vi "CD Shared lvlib.vi"(9 "Action":T1) -> (1 "Output":string)   [LabVIEW 2020, in "NIVS_Consolidated_CDW_MetaDataObj.lvclass"]
doc: "Constants, which are necessary for the <B>CD Shared library</B> in the generated custom device project."
uses:
  NIVS_Consolidated_CDW_MetaDataObj.lvclass
  CD Shared lvlib.ctl
  Common.ctl
  Common.vi
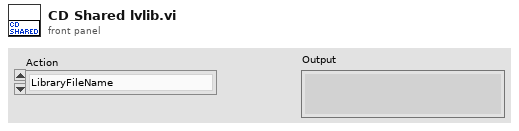
[diagram p1: front panel]
types:
  T1 = typedef "NIVS_Consolidated_CDW_MetaDataObj.lvclass/CD Shared lvlib.ctl" = enum16{"LibraryFileName", "LibraryFolderName", "ConstantsVI.VIPathAndName", "Shared.FolderName", "Shared.Types.FolderName", "Shared.Constants.VIName", "Shared.Constants.VITemplateName", "Shared.Constants.VITemplatePathAndName", "Shared.CompiledSettings.RelativePath", "Shared.Constants.RelativePath", "Shared.CompiledSettings.Name", "Shared.CompiledSettings.Name.NoExtension", "Shared.CompiledSettings.ClusterName"}
  T2 = typedef "NIVS_Consolidated_CDW_MetaDataObj.lvclass/Common.ctl" = enum16{"ProjectName", "TemplatesFolderName", "PPLTemplatesFolderName", "ProjectTemplatePathAndName", "ProjectPPLTemplatePathAndName", "TimingAndSyncFolderName", "CustomDeviceFolderName", "PathToTemplates", "PathToPPLTemplates", "PathToExplorerPPLTemplates", "PathToEnginePPLTemplates", "PathToConfigurationFile", "ProjectConfigurationName"}
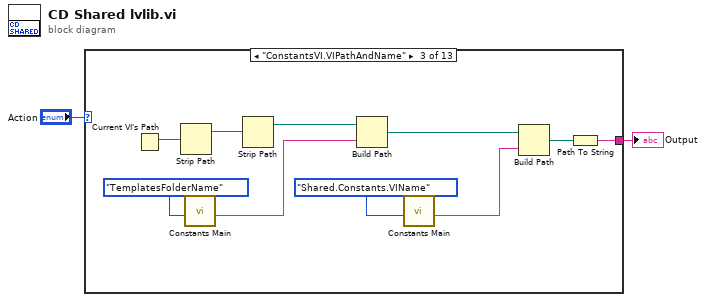
[diagram p0: block diagram]
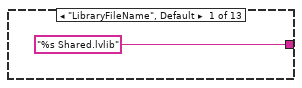
[diagram p2: hidden frame]
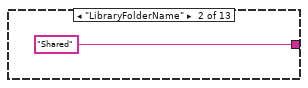
[diagram p3: hidden frame]
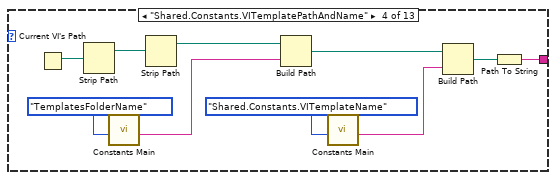
[diagram p4: hidden frame]
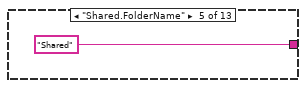
[diagram p5: hidden frame]
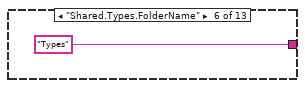
[diagram p6: hidden frame]
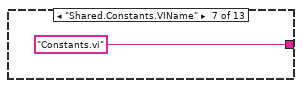
[diagram p7: hidden frame]
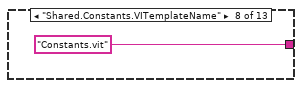
[diagram p8: hidden frame]
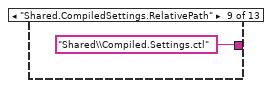
[diagram p9: hidden frame]
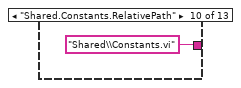
[diagram p10: hidden frame]
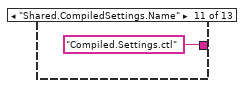
[diagram p11: hidden frame]
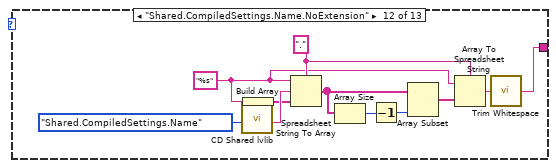
[diagram p12: hidden frame]
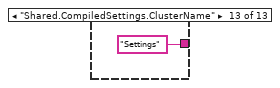
[diagram p13: hidden frame]
diagram:
  n1 = case shown="\"ConstantsVI.VIPathAndName\"" "Action" {
    tunnel: ["%s Shared.lvlib" "Shared" w14 w24 "Shared" "Types" "Constants.vi" "Constants.vit" "Shared\\Compiled.Settings.ctl" ("name or relative path") "Shared\\Constants.vi" ("name or relative path") "Compiled.Settings.ctl" ("name or relative path") w32 "Settings" ("name or relative path")] -> w2
    frame "LibraryFileName", Default {
    }
    frame "LibraryFolderName" {
    }
    frame "ConstantsVI.VIPathAndName" {
      n2 = Current VI's Path() -> (path=w7:path)
      n3 = Strip Path(path=w7) -> (stripped path=w6:path)  [unwired: 1 out]
      n4 = call-poly "Constants Main.vi"("Action"=Common."TemplatesFolderName") -> ("Output"=w12:string)  [unwired: 10 in]
      n5 = Strip Path(path=w6) -> (stripped path=w5:path)  [unwired: 1 out]
      n6 = Build Path(base path=w5, name or relative path=w12) -> (appended path=w11:path)
      n7 = call-poly "Constants Main.vi"("Action"=CD_Shared_lvlib."Shared.Constants.VIName") -> ("Output"=w8:string)  [unwired: 10 in]
      n8 = Build Path(base path=w11, name or relative path=w8) -> (appended path=w10:path)
      n9 = Path To String(path=w10) -> (string=w14:string)
    }
    frame "Shared.Constants.VITemplatePathAndName" {
      n10 = Current VI's Path() -> (path=w17:path)
      n11 = Strip Path(path=w17) -> (stripped path=w16:path)  [unwired: 1 out]
      n12 = call-poly "Constants Main.vi"("Action"=Common."TemplatesFolderName") -> ("Output"=w22:string)  [unwired: 10 in]
      n13 = Strip Path(path=w16) -> (stripped path=w15:path)  [unwired: 1 out]
      n14 = Build Path(base path=w15, name or relative path=w22) -> (appended path=w21:path)
      n15 = call-poly "Constants Main.vi"("Action"=CD_Shared_lvlib."Shared.Constants.VITemplateName") -> ("Output"=w18:string)  [unwired: 10 in]
      n16 = Build Path(base path=w21, name or relative path=w18) -> (appended path=w20:path)
      n17 = Path To String(path=w20) -> (string=w24:string)
    }
    frame "Shared.FolderName" {
    }
    frame "Shared.Types.FolderName" {
    }
    frame "Shared.Constants.VIName" {
    }
    frame "Shared.Constants.VITemplateName" {
    }
    frame "Shared.CompiledSettings.RelativePath" {
    }
    frame "Shared.Constants.RelativePath" {
    }
    frame "Shared.CompiledSettings.Name" {
    }
    frame "Shared.CompiledSettings.Name.NoExtension" {
      w35 = "." ("delimiter (Tab)")
      w34 = "%s" ("format string")
      n18 = call "CD Shared lvlib.vi"("Action"=CD_Shared_lvlib."Shared.CompiledSettings.Name") -> ("Output"=w41:string)  [unwired: 10 in]
      n19 = Build Array(w34) -> (w40:string[])
      n20 = Spreadsheet String To Array(delimiter (Tab)=w35, format string=w34, spreadsheet string=w41, array type (2D Dbl)=w40) -> (array=w39:string[])
      n21 = Array Size(array=w39) -> (size(s)=w38:i32)
      n22 = Decrement(x=w38) -> (x-1=w37:i32)
      n23 = Array Subset(array=w39, length=w37) -> (w36:string[])  [unwired: 1 in]
      n24 = Array To Spreadsheet String(delimiter (Tab)=w35, array=w36, 3:w34) -> (spreadsheet string=w33:string)
      n25 = call <vilib>:"Trim Whitespace.vi"("string"=w33) -> ("trimmed string"=w32:string)  [unwired: 1 in]
    }
    frame "Shared.CompiledSettings.ClusterName" {
    }
  }
  "Output" <- w2
